vi "Actor Core.vi"(8 "error in":errorcluster, 11 "Power Meter in":refnum<class "Power Meter.lvclass">) -> (0 "error out":errorcluster, 3 "Actor out":refnum<class "Actor.lvclass">)   [LabVIEW 2018, in "Power Meter.lvlib" / "Power Meter.lvclass"]
doc: "(<B>Filename</B>: Actor Framework.lvlib:Actor.lvclass:Actor Core.vi)\n\nReceives messages to the actor, reacts to them, and initiates any error handling that may shut the actor down.\n\nDescendant classes may override this VI to append parallel tasks for the actor to complete while it handles messages. Overrides use the Call Parent Method node."
uses:
  Power Meter.lvclass
  C:/Program Files/National Instruments/LabVIEW 2018/vi.lib/ActorFramework/Actor/Actor.lvclass
  <vilib>/ActorFramework/Actor/Actor.lvclass
  Power Meter.lvclass/Power Meter.ctl
  <vilib>/ActorFramework/Actor/Actor.lvclass/Actor.ctl
  <vilib>/ActorFramework/Message Enqueuer/Message Enqueuer.lvclass/Message Enqueuer.ctl
  <vilib>/ActorFramework/Message Enqueuer/Message Priority.ctl
  <vilib>/ActorFramework/Message Enqueuer/Init from Existing Queue.vi
  <vilib>/ActorFramework/Message Enqueuer/Enqueue.vi
  Power Meter Messages/get power Msg/get power Msg.lvclass
  C:/Program Files/National Instruments/LabVIEW 2018/vi.lib/ActorFramework/Message/Message.lvclass
  <vilib>/ActorFramework/Message Priority Queue/Priority Enqueue.vi
  <vilib>/ActorFramework/Message Enqueuer/Message Enqueuer.lvclass
  Device/Device.lvclass
  Power Meter.lvlib
panel:
  in  "Stop Button":bool
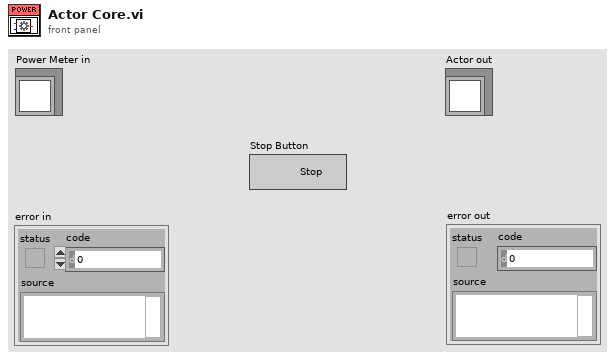
[diagram p1: front panel]
types:
  T1 = typedef "Actor Framework.lvlib/Message Enqueuer.lvclass/Message Priority.ctl" = enum16{"Low", "Normal", "High"}
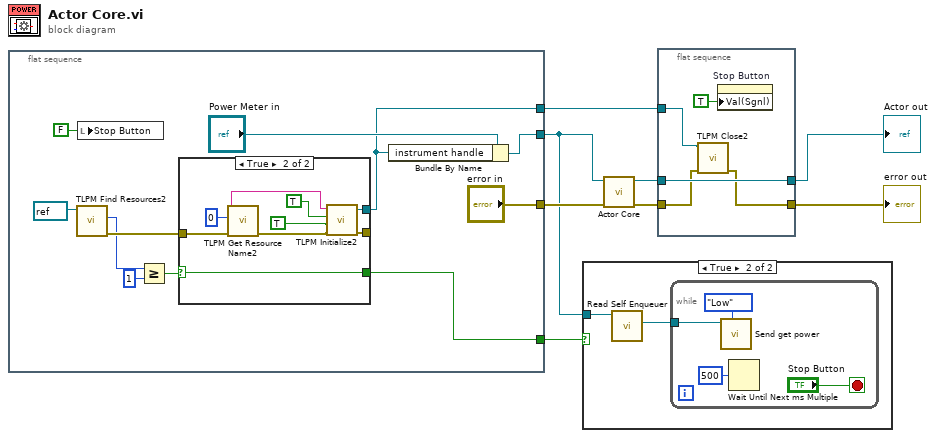
[diagram p0: block diagram]
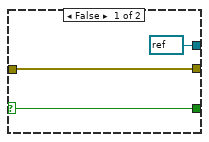
[diagram p3: hidden frame]
diagram:
  n1 = flat-sequence {
    tunnel: ["error in"] -> w8
    tunnel: [w16] -> w7
    tunnel: [w13] -> w2
    tunnel: [w12] -> w1
    frame #0 {
      n2 = call "TLPM Find Resources2.vi"("instrument handle"=refnum<visa-resource-name> refnum) -> ("error out"=w11:errorcluster, "Resource Count"=w10:u32)  [unwired: 8 in, 1 out]
      n3 = local write "Stop Button"(FALSE ("Stop Button")) -> ()
      n4 = Greater Or Equal?(x=w10, y=u32 1) -> (x >= y?=w14:bool)
      n5 = case shown="True" w14 {
        selector: w14 -> [w21 w31]
        tunnel: [refnum<visa-resource-name> refnum ("instrument handle out") w26] -> w13
        tunnel: w11 -> [w20 w30]
        tunnel: [w21 w31] -> w12
        tunnel: [w20 w27] -> _
        frame False {
        }
        frame True {
          n6 = call "TLPM Get Resource Name2.vi"("error in (no error)"=w30, "Index (0)"=u32 0 ("Device Index")) -> ("error out"=w28:errorcluster, "Resource Name"=w23:string)  [unwired: 7 in, 1 out]
          n7 = call "TLPM Initialize2.vi"("error in (no error)"=w28, "Reset Device (Reset Device)"=TRUE ("ID Query (Do Query)"), "ID Query (Do Query)"=TRUE, "resource name"=w23) -> ("error out"=w27:errorcluster, "instrument handle out"=w26:refnum<visa-resource-name>)  [unwired: 6 in]
        }
      }
      n8 = Bundle By Name(cluster="Power Meter in", "instrument handle"=w13) -> (w16:refnum<class "Power Meter.lvclass">)
    }
  }
  n9 = case shown="True" w1 {
    tunnel: w7 -> [_ w33]
    frame False {
    }
    frame True {
      n10 = call <vilib>:"Read Self Enqueuer.vi"("Actor"=w33) -> ("Self Enqueuer"=w32:refnum<class "Message Enqueuer.lvclass">)  [unwired: 10 in]
      n11 = while {
        tunnel: w32 -> [w35]
        stop <- "Stop Button" stop-if-true
        n12 = call "Send get power.vi"("Message Priority (Normal)"=Message_Priority."Low", "Message Enqueuer"=w35) -> ()  [unwired: 8 in, 2 out]
        n13 = Wait Until Next ms Multiple(millisecond multiple=u32 500) -> ()  [unwired: 1 out]
      }
    }
  }
  n14 = call-parent "Actor Core.vi"("error in"=w8, "Device in"=w7) -> ("error out"=w4:errorcluster, "Actor out"=w6:refnum<class "Actor.lvclass">)  [unwired: 8 in]
  n15 = flat-sequence {
    tunnel: w6 -> [w42]
    tunnel: [w42] -> w5
    tunnel: w4 -> [w39]
    tunnel: [w38] -> w3
    tunnel: w2 -> [w40]
    frame #0 {
      n16 = call "TLPM Close2.vi"("error in (no error)"=w39, "instrument handle"=w40) -> ("error out"=w38:errorcluster)  [unwired: 9 in]
      n17 = property on="Stop Button" class="Bool (strict)"("Val(Sgnl)"=TRUE ("Value (Signaling)")) -> ()  [unwired: 2 in, 2 out]
    }
  }
  "error out" <- w3
  "Actor out" <- w5
